vi "Trigger FXP(+,-,18,1).vi"(0 "data A":fxp<+/-,18,1>[](array[numeric])=[0.0, 0.0], 1 "reset":bool, 2 "trigger.ready for reference":bool, 5 "data B":fxp<+/-,18,1>[](array[numeric])=[0.0, 0.0], 7 "input valid":bool, 9 "trigger.A":T8, 11 "trigger.B":T7, 12 "trigger.combination type":T10=enum."A", 13 "rearm delay":u16=2) -> (4 "timestamps":T1, 6 "trigger.out":T9, 8 "overflow":bool)   [LabVIEW 2021]
uses:
  FPGA Interface Typedefinitions/Trigger Combination Type.ctl
  <instrlib>/_niInstr/Types/v1/Shared/Public/Input Triggers.ctl
  SubVIs/Types/Trigger Type.ctl
  <instrlib>/_niInstr/Data Trigger/v1/Shared/Public/Level Configuration FXP(+-,18,1).ctl
  <instrlib>/_niInstr/Data Trigger/v1/Shared/Public/Level Configuration Trigger When.ctl
  <instrlib>/_niInstr/Data Trigger/v1/Shared/Public/Edge Configuration FXP(+-,18,1).ctl
  <instrlib>/_niInstr/Data Trigger/v1/Shared/Public/Edge Configuration Trigger Slope.ctl
  <instrlib>/_niInstr/Multirecord Acquisition/Interface/v1/FPGA/Public/Timestamp.ctl
  <instrlib>/_niInstr/Data Trigger/v1/FPGA/Private/Trigger/Level FXP(+-,18,1)xNspc.vi
  <instrlib>/_niInstr/Data Trigger/v1/FPGA/Private/Trigger/Edge FXP(+-,18,1)xNspc.vi
  Trigger Interpolation/Trigger Interpolation FXP(+,-,18,1)x2spc.vi
  <instrlib>/_niInstr/Basic Elements/v1/FPGA/Private/D Latch U16.vi
  <instrlib>/_niInstr/Types/v1/Shared/niInstr Types v1 Shared.lvlib
  <instrlib>/_niInstr/Basic Elements/v1/FPGA/niInstr Basic Elements v1 FPGA.lvlib
  <instrlib>/_niInstr/Data Trigger/v1/FPGA/niInstr Data Trigger v1 FPGA.lvlib
  <instrlib>/_niInstr/Multirecord Acquisition/Interface/v1/FPGA/niInstr Multirecord Acquisition v1 FPGA.lvclass
  <instrlib>/_niInstr/Data Trigger/v1/Shared/niInstr Data Trigger v1 Shared.lvlib
  FPGA Interface Typedefinitions/FPGA Interface Typedefinitions.lvlib
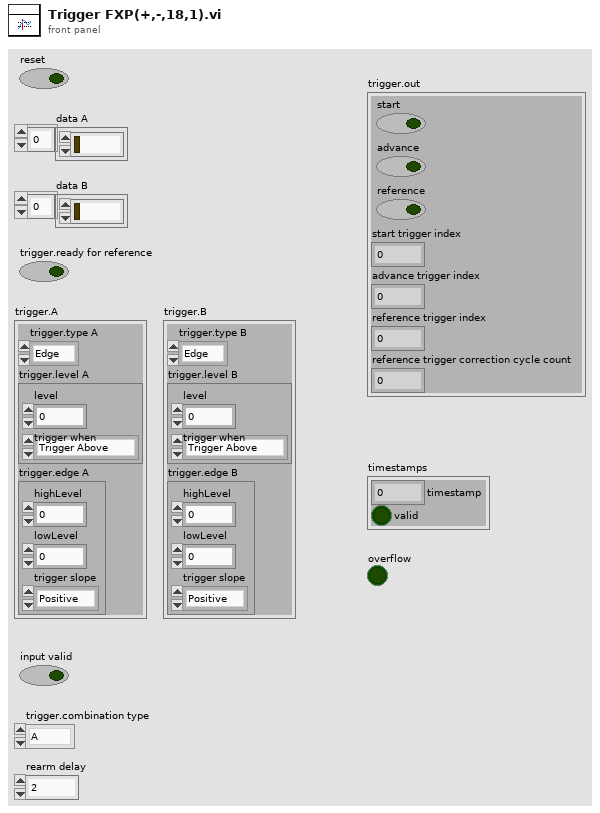
[diagram p1: front panel]
types:
  T1 = typedef "niInstr Multirecord Acquisition v1 FPGA.lvclass/Timestamp.ctl" = cluster{"timestamp":u64, "valid":bool}
  T2 = typedef "Trigger Type.ctl" = enum16{"Edge", "Level", "Custom"}
  T3 = typedef "niInstr Data Trigger v1 Shared.lvlib/Level Configuration FXP(+-,18,1).ctl" = cluster{"level":fxp<+/-,18,1>, "trigger when":T4}
  T4 = typedef "niInstr Data Trigger v1 Shared.lvlib/Level Configuration Trigger When.ctl" = enum8{"Trigger Above", "Trigger Below"}
  T5 = typedef "niInstr Data Trigger v1 Shared.lvlib/Edge Configuration FXP(+-,18,1).ctl" = cluster{"highLevel":fxp<+/-,18,1>, "lowLevel":fxp<+/-,18,1>, "trigger slope":T6}
  T6 = typedef "niInstr Data Trigger v1 Shared.lvlib/Edge Configuration Trigger Slope.ctl" = enum8{"Positive", "Negative"}
  T7 = cluster{"trigger.type B":T2, "trigger.level B":T3, "trigger.edge B":T5}
  T8 = cluster{"trigger.type A":T2, "trigger.level A":T3, "trigger.edge A":T5}
  T9 = typedef "niInstr Types v1 Shared.lvlib/Input Triggers.ctl" = cluster{"start":bool, "advance":bool, "reference":bool, "start trigger index":u16, "advance trigger index":u16, "reference trigger index":u16, "reference trigger correction cycle count":u32}
  T10 = typedef "FPGA Interface Typedefinitions.lvlib/Trigger Combination Type.ctl" = enum16{"Immediate", "A", "B", "OR", "AND", "A THEN B", "B THEN A", "High Resolution"}
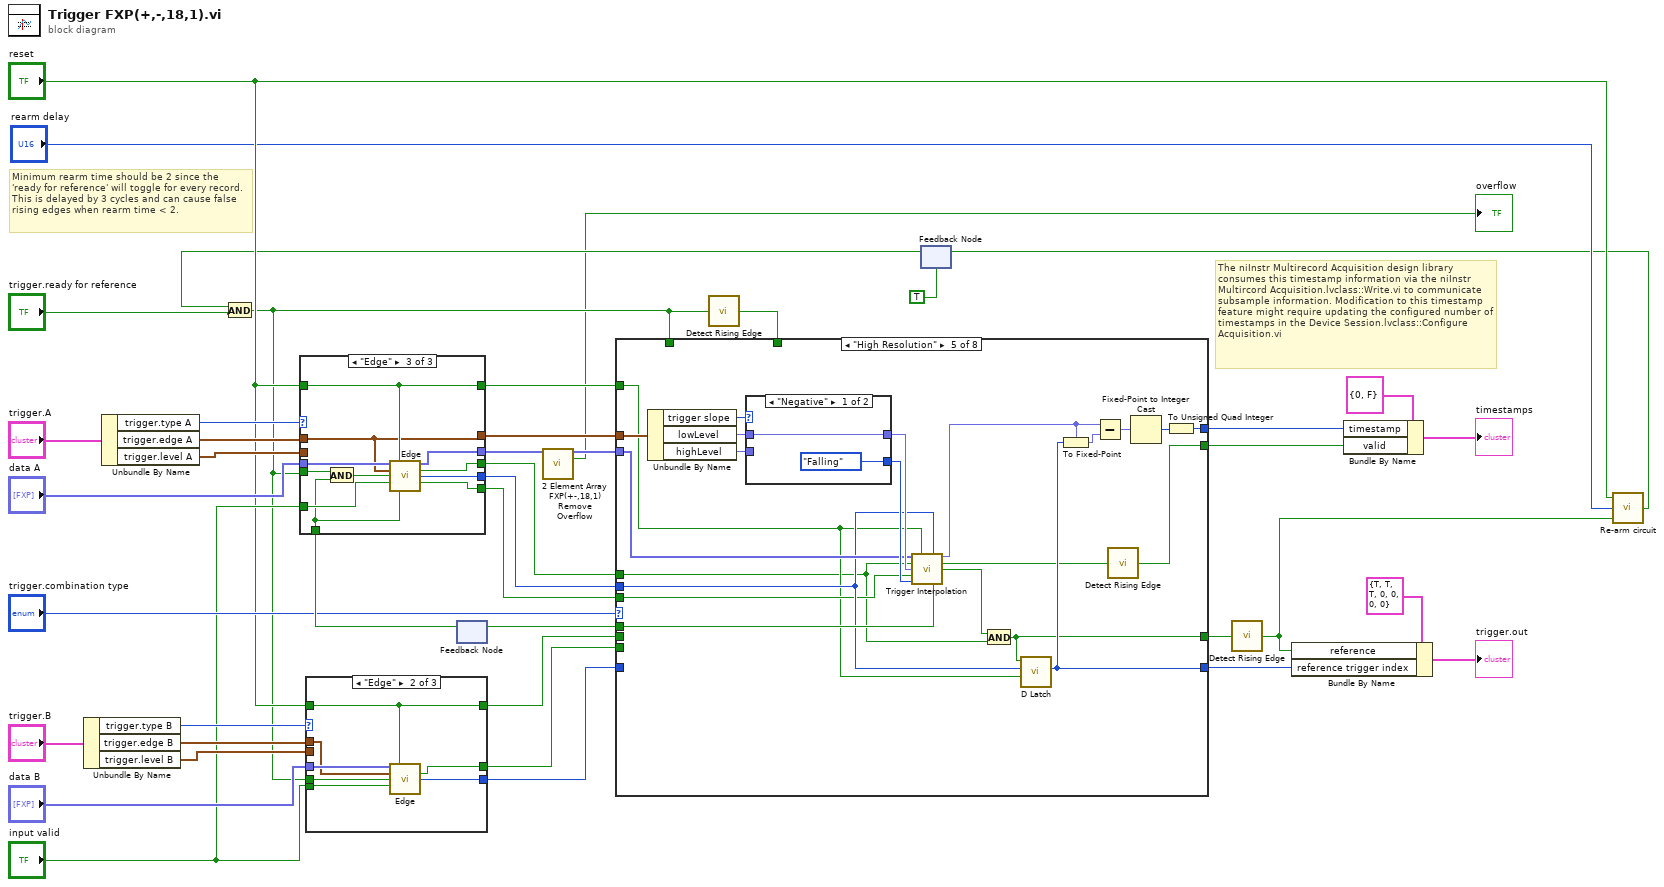
[diagram p0: block diagram]
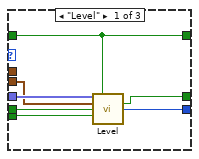
[diagram p2: hidden frame]
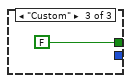
[diagram p3: hidden frame]
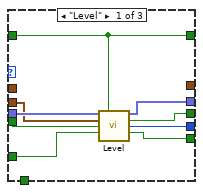
[diagram p4: hidden frame]
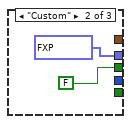
[diagram p5: hidden frame]
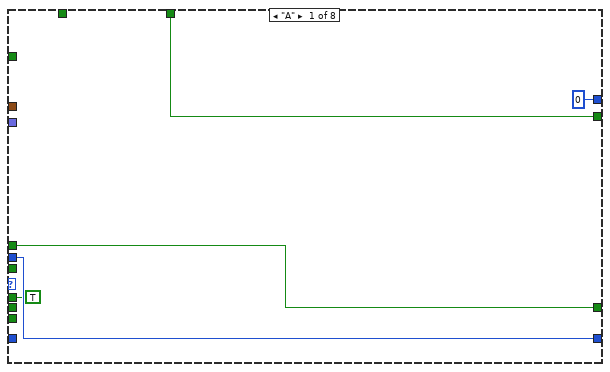
[diagram p6: hidden frame]
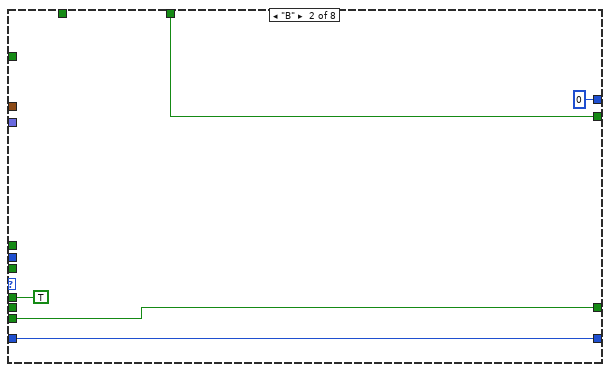
[diagram p7: hidden frame]
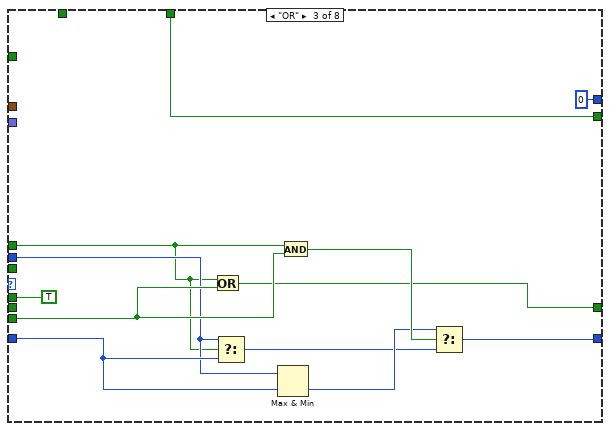
[diagram p8: hidden frame]
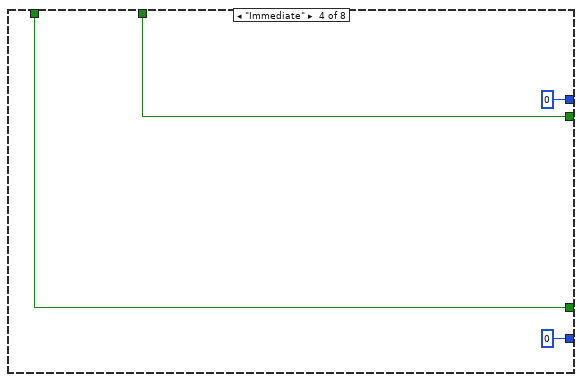
[diagram p9: hidden frame]
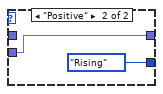
[diagram p10: hidden frame]
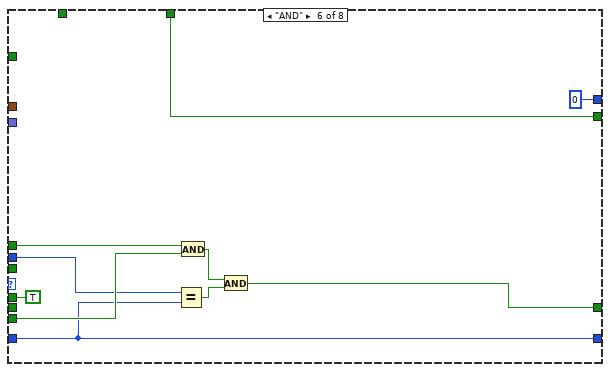
[diagram p11: hidden frame]
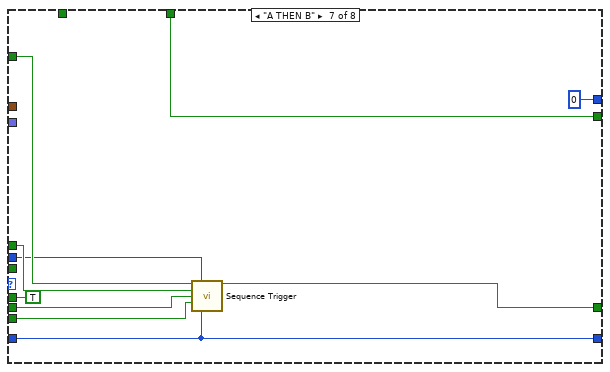
[diagram p12: hidden frame]
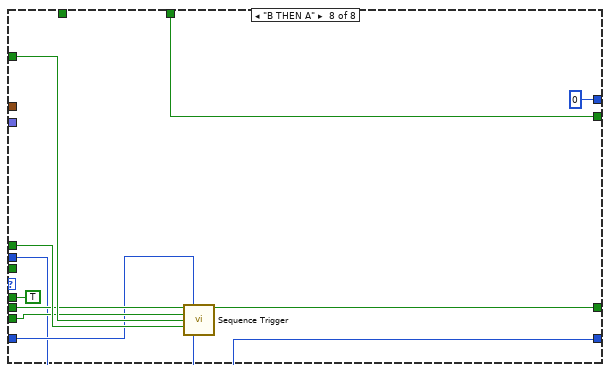
[diagram p13: hidden frame]
diagram:
  # "Minimum rearm time should be 2 since the 'ready for reference' will toggle for every record. This is delayed by 3 cycles and can cause false rising edges when rearm time < 2."
  # "The niInstr Multirecord Acquisition design library consumes this timestamp information via the niInstr Multircord Acquisition.lvclass::Write.vi to communicate subsample information. Modification to this timestamp feature might require updating the configured number of timestamps in the Device Session.lvclass::Configure Acquisition.vi"
  n1 = Unbundle By Name("trigger.B") -> ("trigger.type B"=w23:T2, "trigger.edge B"=w21:T5, "trigger.level B"=w22:T3)
  n2 = Unbundle By Name("trigger.A") -> ("trigger.type A"=w24:T2, "trigger.edge A"=w26:T5, "trigger.level A"=w27:T3)
  n3 = feedback #1() -> (w40:bool)  [unwired: 1 in]
  n4 = feedback #2(TRUE ("rearm out")) -> (w5:bool)
  n5 = And(x=w5, y="trigger.ready for reference") -> (x .and. y?=w4:bool)
  n6 = case shown="\"Edge\"" w24 {
    tunnel: "input valid" -> [w51 _ w64]
    tunnel: [w50 FALSE ("trigger") w63] -> w30
    tunnel: [w49 _ w62] -> w33
    tunnel: [w47 _ w60] -> w37
    tunnel: "data A" -> [w48 _ w61]
    tunnel: "reset" -> [w47 _ w60]
    tunnel: [w46 _ w59] -> w39
    tunnel: w4 -> [w44 _ w56]
    tunnel: [_ _ w57] -> w38
    tunnel: [w45 fxp<+/-,18,1>[] [0.0, 0.0] ("data out") w58] -> w3
    tunnel: w40 -> [_ _ w54]
    tunnel: w26 -> [_ _ w57]
    tunnel: w27 -> [w43 _ _]
    frame "Level" {
      n7 = call-poly <instrlib>:"Level.vi"("data in"=w48, "reset"=w47, "configuration"=w43, "arm (T)"=w44, "input valid"=w51) -> ("data out"=w45:fxp<+/-,18,1>[], "trigger"=w50:bool, "trigger index"=w49:u16, "output valid"=w46:bool)  [unwired: 5 in, 2 out]
    }
    frame "Custom" {
    }
    frame "Edge" {
      n8 = And(x=w56, y=w54) -> (x .and. y?=w55:bool)
      n9 = call-poly <instrlib>:"Edge.vi"("data in"=w61, "reset"=w60, "configuration"=w57, "arm (T)"=w55, "input valid"=w64, "ready for output (T)"=w54) -> ("data out"=w58:fxp<+/-,18,1>[], "trigger"=w63:bool, "trigger index"=w62:u16, "output valid"=w59:bool)  [unwired: 4 in, 2 out]
    }
  }
  n10 = case shown="\"Edge\"" w23 {
    tunnel: [w71 w78 FALSE ("trigger")] -> w31
    tunnel: "input valid" -> [w70 w77 _]
    tunnel: [w69 w76 _] -> w34
    tunnel: [w67 w74 _] -> w35
    tunnel: "data B" -> [w68 w75 _]
    tunnel: "reset" -> [w67 w74 _]
    tunnel: w22 -> [w66 _ _]
    tunnel: w21 -> [_ w73 _]
    tunnel: w4 -> [w65 w72 _]
    frame "Level" {
      n11 = call-poly <instrlib>:"Level.vi"("data in"=w68, "reset"=w67, "configuration"=w66, "arm (T)"=w65, "input valid"=w70) -> ("trigger"=w71:bool, "trigger index"=w69:u16)  [unwired: 5 in, 4 out]
    }
    frame "Edge" {
      n12 = call-poly <instrlib>:"Edge.vi"("data in"=w75, "reset"=w74, "configuration"=w73, "arm (T)"=w72, "input valid"=w77) -> ("trigger"=w78:bool, "trigger index"=w76:u16)  [unwired: 5 in, 4 out]
    }
    frame "Custom" {
    }
  }
  n13 = call "2 Element Array FXP(+-,18,1) Remove Overflow.vi"("data in"=w3) -> ("data out"=w2:fxp<+/-,18,1>[], "overflow"=→"overflow":bool)  [unwired: 13 in]
  n14 = call <instrlib>:"Detect Rising Edge.vi"("signal"=w4) -> ("edge detected"=w13:bool)  [unwired: 14 in]
  n15 = case shown="\"High Resolution\"" "trigger.combination type" {
    tunnel: w30 -> [w84 _ w93 _ w108 w141 w150 w159]
    tunnel: w31 -> [_ w89 w95 _ _ w140 w148 w158]
    tunnel: [w84 w89 w92 w103 w106 w136 w147 w161] -> w12
    tunnel: w33 -> [w83 _ w94 _ w113 w139 w143 w152]
    tunnel: w34 -> [_ w88 w96 _ _ w135 w142 w153]
    tunnel: [w83 w88 w91 u16 0 ("trigger index") w115 w135 w142 w152] -> w36
    tunnel: w37 -> [_ _ _ _ w109 _ w151 w160]
    tunnel: w35 -> [_ _ _ _ _ _ w149 w157]
    tunnel: w38 -> [_ _ _ _ w126 _ _ _]
    tunnel: w2 -> [_ _ _ _ w114 _ _ _]
    tunnel: w39 -> [_ _ _ _ w112 _ _ _]
    tunnel: [u64 0 ("trigger time") u64 0 ("trigger time") u64 0 ("trigger time") u64 0 ("trigger time") w124 u64 0 ("trigger time") u64 0 ("trigger time") u64 0 ("trigger time")] -> w20
    tunnel: [w80 w85 w100 w102 w110 w132 w144 w154] -> w19
    tunnel: w4 -> [_ _ _ w103 _ _ _ _]
    tunnel: [TRUE ("ready for input") TRUE ("ready for input") TRUE ("ready for input") _ w122 TRUE ("ready for input") TRUE ("ready for input") TRUE ("ready for input")] -> w41
    tunnel: w13 -> [w80 w85 w100 w102 _ w132 w144 w154]
    frame "A" {
    }
    frame "B" {
    }
    frame "OR" {
      n16 = Or(x=w93, y=w95) -> (x .or. y?=w92:bool)
      n17 = Select(t=w94, s=w93, f=w96) -> (s? t:f=w97:u16)
      n18 = Max & Min(x=w94, y=w96) -> (min(x,y)=w98:u16)  [unwired: 1 out]
      n19 = And(x=w93, y=w95) -> (x .and. y?=w99:bool)
      n20 = Select(t=w98, s=w99, f=w97) -> (s? t:f=w91:u16)
    }
    frame "Immediate" {
    }
    frame "High Resolution" {
      n21 = Unbundle By Name(w126) -> ("trigger slope"=w123:T6, "lowLevel"=w120:fxp<+/-,18,1>, "highLevel"=w119:fxp<+/-,18,1>)
      n22 = case shown="\"Negative\"" w123 {
        tunnel: [enum16{"Rising", "Falling"}."Falling" ("trigger direction") enum16{"Rising", "Falling"}."Rising" ("trigger direction")] -> w127
        tunnel: [w128 w130] -> w121
        tunnel: w120 -> [w128 _]
        tunnel: w119 -> [_ w130]
        frame "Negative" {
        }
        frame "Positive" {
        }
      }
      n23 = call-poly "Trigger Interpolation.vi"("data in"=w114, "reset"=w109, "trigger index"=w113, "trigger"=w108, "trigger level"=w121, "data valid"=w112, "trigger direction"=w127) -> ("trigger time"=w117:fxp<+/-,32,5>, "trigger time valid"=w111:bool, "ready for trigger"=w107:bool, "ready for input"=w122:bool)  [unwired: 4 in, 1 out]
      n24 = And(x=w107, y=w108) -> (x .and. y?=w106:bool)
      n25 = call-poly <instrlib>:"D Latch.vi"("r"=w109, "d"=w113, "s"=w106) -> ("q"=w115:u16)  [unwired: 8 in]
      n26 = To Fixed-Point(fixed-point type=w117, number=w115) -> (fixed-point=w118:fxp<+/-,32,5>)
      n27 = Subtract(x=w117, y=w118) -> (x-y=w116:fxp<+/-,33,6>)
      n28 = call <instrlib>:"Detect Rising Edge.vi"("signal"=w111) -> ("edge detected"=w110:bool)  [unwired: 14 in]
      n29 = Fixed-Point to Integer Cast(1:w116) -> (0:w125:i64)
      n30 = To Unsigned Quad Integer(1:w125) -> (0:w124:u64)
    }
    frame "AND" {
      n31 = Equal?(x=w139, y=w135) -> (x = y?=w137:bool)
      n32 = And(x=w141, y=w140) -> (x .and. y?=w138:bool)
      n33 = And(x=w138, y=w137) -> (x .and. y?=w136:bool)
    }
    frame "A THEN B" {
      n34 = call "Sequence Trigger.vi"("reset A"=w151, "trigger index A"=w143, "A"=w150, "reset B"=w149, "B"=w148, "trigger index B"=w142) -> ("trigger"=w147:bool)  [unwired: 9 in]
    }
    frame "B THEN A" {
      n35 = call "Sequence Trigger.vi"("reset A"=w157, "trigger index A"=w153, "A"=w158, "reset B"=w160, "B"=w159, "trigger index B"=w152) -> ("trigger"=w161:bool)  [unwired: 9 in]
    }
  }
  n36 = feedback-in #1(w41) -> ()
  n37 = call <instrlib>:"Detect Rising Edge.vi"("signal"=w12) -> ("edge detected"=w11:bool)  [unwired: 14 in]
  n38 = Bundle By Name(cluster=T9 {"start"=TRUE, "advance"=TRUE, "reference"=TRUE, "start trigger index"=0, "advance trigger index"=0, "reference trigger index"=0, "reference trigger correction cycle count"=0} ("triggers in"), "reference"=w11, "reference trigger index"=w36) -> (→"trigger.out":T9)
  n39 = Bundle By Name(cluster=T1 {"timestamp"=0, "valid"=FALSE} ("timestamp"), "timestamp"=w20, "valid"=w19) -> (→"timestamps":T1)
  n40 = call "Re-arm circuit.vi"("trigger"=w11, "delay"="rearm delay", "reset"="reset") -> ("rearm out"=w8:bool)
  n41 = feedback-in #2(w8) -> ()
